vi "main.vi"() -> ()   [LabVIEW 2020]
uses:
  ctl/9-id,name,path.ctl
  ctl/0-id,name.ctl
  ctl/7-id,name,fields.ctl
panel:
  out "items":T1[](array[typedef]) {"int 3" format="%.0x"; "size" format="%.0x"}
  out "list":T2[](array[typedef])
  out "root elems":T3[](array[typedef])
  out "error out":errorcluster
  out "data out":string
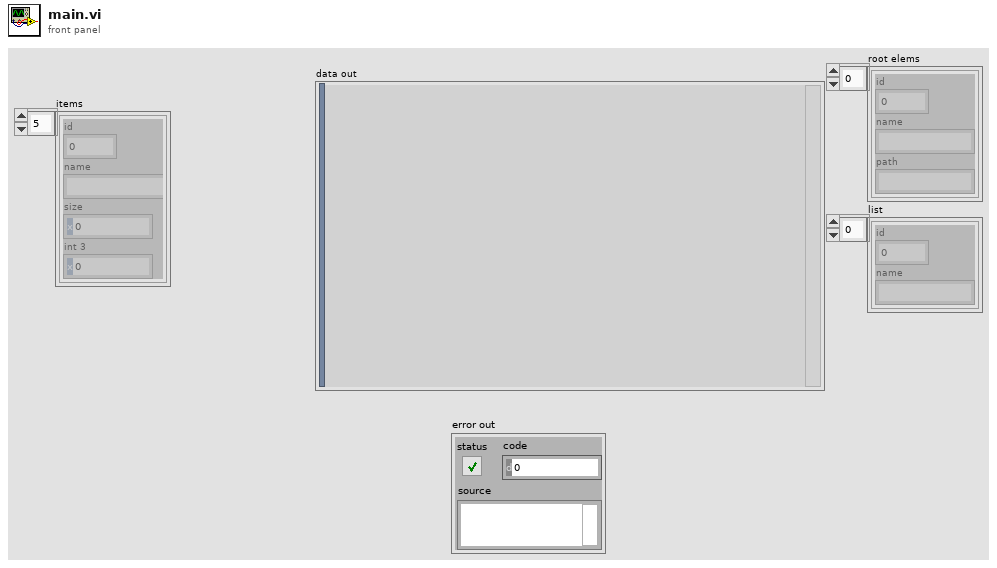
[diagram p1: front panel]
types:
  T1 = typedef "7-id,name,fields.ctl" = cluster{"id":i16, "name":string, "size":u64, "int 3":u32}
  T2 = typedef "0-id,name.ctl" = cluster{"id":u8, "name":string}
  T3 = typedef "9-id,name,path.ctl" = cluster{"id":u8, "name":string, "path":string}
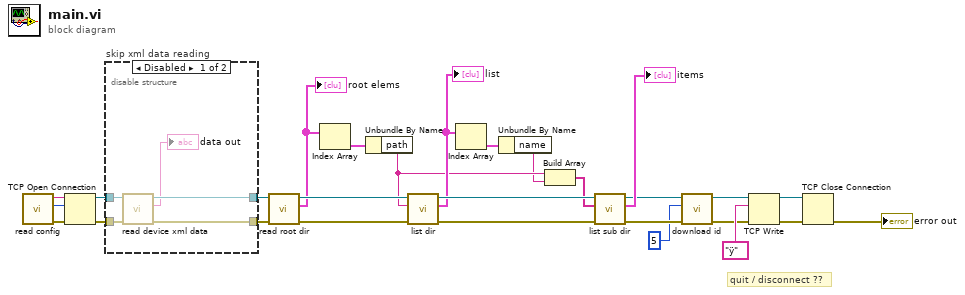
[diagram p0: block diagram]
diagram:
  # "quit / disconnect ??"
  n1 = call "read config.vi"() -> ("error out"=w1:errorcluster, "port"=w2:i32, "host"=w3:string)  [unwired: 9 in]
  n2 = TCP Open Connection(address=w3, remote port or service name=w2, error in (no error)=w1) -> (connection ID=w28:refnum<k5>, error out=w27:errorcluster)  [unwired: 2 in]
  n3 = disable-structure "skip xml data reading" shown="Disabled" {
    disable-tunnel: w28 -> [w33 w35]
    disable-tunnel: w27 -> [w32 w34]
    disable-tunnel: [w31 w34] -> w22
    disable-tunnel: [w30 w35] -> w21
    frame Disabled {
      n4 = call "read device xml data.vi"("error in (no error)"=w32, "TCP Network Connection in"=w33) -> ("error out"=w31:errorcluster, "data out"=→"data out":string, "TCP Network Connection out"=w30:refnum<k5>)  [unwired: 7 in]
    }
    frame Enabled {
    }
  }
  n5 = call "read root dir.vi"("error in (no error)"=w22, "TCP in"=w21) -> ("error out"=w20:errorcluster, "root elements"=w18:T3[], "TCP out"=w19:refnum<k5>)  [unwired: 7 in]
  "root elems" <- w18
  n6 = Index Array(array=w18) -> (element=w17:T3)  [unwired: 1 in]
  n7 = Unbundle By Name(w17) -> ("path"=w12:string)
  n8 = call "list dir.vi"("error in (no error)"=w20, "path"=w12, "TCP in"=w19) -> ("error out"=w16:errorcluster, "Array"=w13:T2[], "TCP out"=w15:refnum<k5>)  [unwired: 6 in]
  "list" <- w13
  n9 = Index Array(array=w13) -> (element=w14:T2)  [unwired: 1 in]
  n10 = Unbundle By Name(w14) -> ("name"=w11:string)
  n11 = Build Array(w12, w11) -> (w10:string[])
  n12 = call "list sub dir.vi"("error in (no error)"=w16, "path items"=w10, "TCP in"=w15) -> ("error out"=w8:errorcluster, "Array"=→"items":T1[], "TCP out"=w6:refnum<k5>)  [unwired: 6 in]
  n13 = call "download id.vi"("error in (no error)"=w8, "id"=i16 5, "TCP in"=w6) -> ("error out"=w7:errorcluster, "TCP out"=w5:refnum<k5>)  [unwired: 7 in]
  n14 = TCP Write(connection ID=w5, data in="ÿ", error in (no error)=w7) -> (connection ID out=w24:refnum<k5>, error out=w25:errorcluster)  [unwired: 1 in, 1 out]
  n15 = TCP Close Connection(connection ID=w24, error in (no error)=w25) -> (error out=→"error out":errorcluster)  [unwired: 1 in, 1 out]
